vi "Evaluate Polynomial with Matrix (CDB).vi"(2 "P(x)":cdb[](array[numeric]) format="%#.6g", 3 "A":T1) -> (0 "error":i32, 1 "P([A])":T1)   [LabVIEW 2014, in "NI_AALPro.lvlib"]
doc: "Evaluates the polynomial <B>P(x)</B> with matrix <B>A</B>. The data types you wire to the <B>P(x)</B> and <B>A</B> inputs determine the polymorphic instance to use."
uses:
  NI_AALPro.lvlib
  ComplexMatrix.ctl
  Complex A x B.vi
  Create Special Complex Matrix.vi
  Multiply - CM,C.vi
  Add - CM,CM.vi
  NI_AALBase.lvlib
  NI_Matrix.lvlib
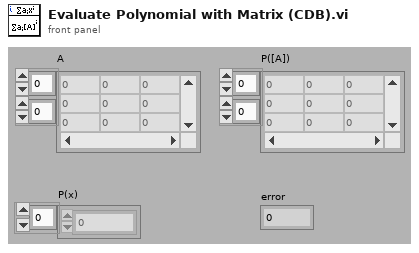
[diagram p1: front panel]
types:
  T1 = typedef "NI_Matrix.lvlib/ComplexMatrix.ctl" = cdb[][]
  T2 = enum32{"Identity", "Diagonal", "Toepliz", "Vandermonde", "Companion"}
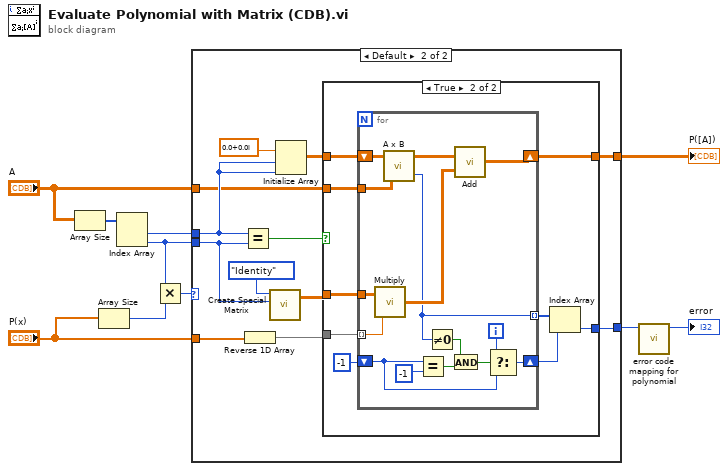
[diagram p0: block diagram]
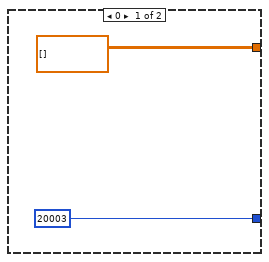
[diagram p2: hidden frame]
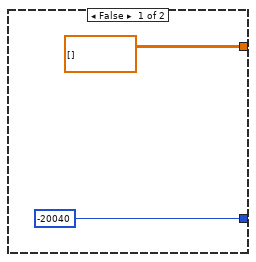
[diagram p3: hidden frame]
diagram:
  n1 = Array Size(array="A") -> (size(s)=w6:i32[])
  n2 = Array Size(array="P(x)") -> (size(s)=w5:i32)
  n3 = Index Array(array=w6) -> (element #1=w10:i32, element #2=w3:i32)  [unwired: 2 in]
  n4 = Multiply(x=w3, y=w5) -> (x*y=w4:i32)
  n5 = case shown="Default" w4 {
    tunnel: w10 -> [_ w22]
    tunnel: [20003 ("empty array") w13] -> w2
    tunnel: "A" -> [_ w17]
    tunnel: "P(x)" -> [_ w16]
    tunnel: [T1 [] ("A") w15] -> w8
    tunnel: w3 -> [_ w14]
    frame 0 {
    }
    frame Default {
      n6 = Equal?(x=w22, y=w14) -> (x = y?=w23:bool)
      n7 = Reverse 1D Array(array=w16) -> (reversed array=w24:cdb[])
      n8 = call-poly "Create Special Matrix.vi"("matrix type"=T2."Identity", "matrix size"=w14) -> ("Special Matrix"=w19:T1)  [unwired: 3 in, 1 out]
      n9 = Initialize Array(cdb 0.0+0.0i, w22, w22) -> (w20:cdb[][])
      n10 = case shown="True" w23 {
        tunnel: w24 -> [_ w35]
        tunnel: w20 -> [_ w34]
        tunnel: w17 -> [_ w33]
        tunnel: w19 -> [_ w32]
        tunnel: [T1 [] ("A") w31] -> w15
        tunnel: [-20040 ("not a square matrix") w27] -> w13
        frame False {
        }
        frame True {
          n11 = for {
            shift-right: [w44] -> w31
            shift-left: w34 -> [w50]
            tunnel: w35 -> [w47] mode=indexing
            tunnel: w33 -> [w49]
            tunnel: w32 -> [w48]
            shift-right: [w36] -> w28
            shift-left: -1 -> [w37]
            tunnel: [w38] -> w29 mode=indexing
            i -> [w39]
            n12 = call-poly "Multiply.vi"("Complex Scalar c"=w47, "Complex Matrix A"=w48) -> ("A * c"=w46:T1)
            n13 = call-poly "A x B.vi"("B"=w49, "A"=w50) -> ("error"=w38:i32, "A x B"=w45:T1)
            n14 = Equal?(x=w37, y=-1) -> (x = y?=w41:bool)
            n15 = Not Equal To 0?(x=w38) -> (x != 0?=w42:bool)
            n16 = And(x=w42, y=w41) -> (x .and. y?=w40:bool)
            n17 = call-poly "Add.vi"("Complex Matrix B"=w46, "Complex Matrix A"=w45) -> ("A + B"=w44:T1)
            n18 = Select(t=w39, s=w40, f=w37) -> (s? t:f=w36:i32)
          }
          n19 = Index Array(array=w29, index=w28) -> (element=w27:i32)
        }
      }
    }
  }
  "P([A])" <- w8
  n20 = call "error code mapping for polynomial.vi"("error in"=w2) -> ("error out"=→"error":i32)  [unwired: 10 in]
